vi "Generate3DTest.vi"(8 "error in (no error)":errorcluster, 11 "Local":T6={"Parameter"={"3D Plot"=[], "3D Scatter"=refnum, "Data"={"Split"={"X Train"=[], "X Test"=[], "Y Train"=[], "Y Test"=[]}, "Predict"=[]}, "Display"={"Choice"=enum."All", "Indexe"={"X"=0, "Y"=1, "Z"=2}}, "Point Property"={"Train Style"=enum."Full circle", "Test OK Style"=enum."Full square", "Label Color"=[8978528, 4367871, 1985280], "Test NO OK"={"Style"=enum."Cross", "Color"=16716800}}, "3D Plot Datatype.lvclass"=refnum}, "3DArray"=[], "Rating 3D Array"=[], "GoodPredict"=0, "Point ID"=[]}) -> (0 "error out":errorcluster, 3 "Local Out":T6)   [LabVIEW 2020]
doc: "Generate the 3D graph with preticted data"
uses:
  _Controls/3DParameters.ctl
  <vilib>/Math Plots/3D Math Plots/3D Plot/3D Plot Datatype/3D Plot Datatype.lvclass
  <vilib>/Math Plots/3D Math Plots/3D Scatter/3D Scatter XCtrl/3D Scatter.xctl
  _Controls/Datas.ctl
  _Controls/PointPropertyMultipleLabel.ctl
  _Controls/Style.ctl
  _Controls/3DData.ctl
types:
  T1 = typedef "3DParameters.ctl" = cluster{"3D Plot":refnum<class "3D Plot Datatype.lvclass">[], "3D Scatter":refnum<vi>, "Data":T2, "Display":cluster{"Choice":enum16{"All", "Train", "Test"}, "Indexe":cluster{"X":i32, "Y":i32, "Z":i32}}, "Point Property":T3, "3D Plot Datatype.lvclass":refnum<class "3D Plot Datatype.lvclass">}
  T2 = typedef "Datas.ctl" = cluster{"Split":cluster{"X Train":dbl[][], "X Test":dbl[][], "Y Train":dbl[][], "Y Test":dbl[][]}, "Predict":dbl[][]}
  T3 = typedef "PointPropertyMultipleLabel.ctl" = cluster{"Train Style":T4, "Test OK Style":T4, "Label Color":u32[], "Test NO OK":cluster{"Style":T4, "Color":u32}}
  T4 = typedef "Style.ctl" = enum16{"Empty circle", "Full circle", "Empty square", "Full square", "Cross"}
  T5 = typedef "3DData.ctl" = cluster{"Tag":i32, "X":dbl[], "Y":dbl[], "Z":dbl[]}
  T6 = cluster{"Parameter":T1, "3DArray":cluster{"X":dbl[], "Y":dbl[], "Z":dbl[]}[], "Rating 3D Array":T5[], "GoodPredict":i32, "Point ID":cluster{"DataUse":enum16{"Dataset", "Train", "Test"}, "Color":u32}[]}
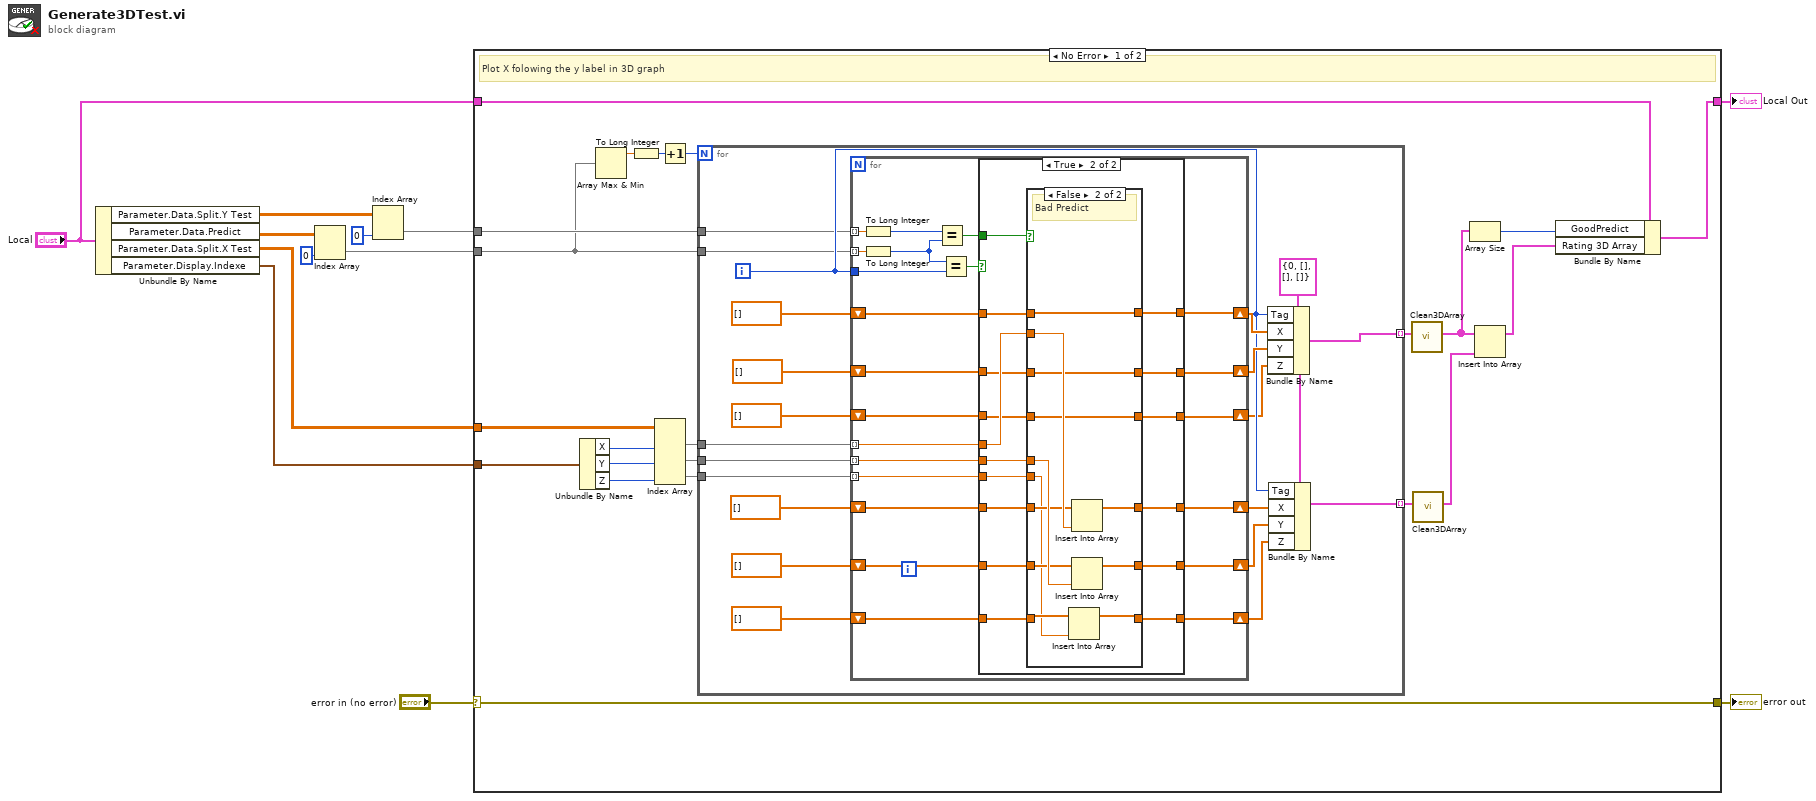
[diagram p0: block diagram]
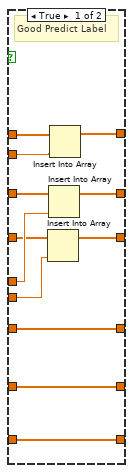
[diagram p3: hidden frame]
diagram:
  n1 = Unbundle By Name("Local") -> ("Parameter.Data.Split.Y Test"=w8:dbl[][], "Parameter.Data.Predict"=w9:dbl[][], "Parameter.Data.Split.X Test"=w5:dbl[][], "Parameter.Display.Indexe"=w3:cluster{"X":i32, "Y":i32, "Z":i32})
  n2 = Index Array(array=w9, index (col)=0 ("disabled index (col)")) -> (element=w6:dbl[])  [unwired: 1 in]
  n3 = Index Array(array=w8, index (col)=0 ("disabled index (col)")) -> (element=w7:dbl[])  [unwired: 1 in]
  n4 = case shown="No Error" "error in (no error)" {
    selector: "error in (no error)" -> [w14 w125]
    tunnel: w5 -> [w32 _]
    tunnel: w6 -> [w24 _]
    tunnel: [w14 w125] -> w12
    tunnel: w7 -> [w25 _]
    tunnel: "Local" -> [w29 w124]
    tunnel: [w28 w124] -> w1
    tunnel: w3 -> [w27 _]
    frame No Error {
      # "Plot X folowing the y label in 3D graph"
      n5 = Unbundle By Name(w27) -> ("X"=w31:i32, "Y"=w30:i32, "Z"=w26:i32)
      n6 = Array Max & Min(array=w24) -> (max value=w34:dbl)  [unwired: 3 out]
      n7 = To Long Integer(number=w34) -> (32bit integer=w33:i32)
      n8 = Index Array(array=w32, index (col) #1=w31, index (col) #2=w30, index (col) #3=w26) -> (element #1=w22:dbl[], element #2=w21:dbl[], element #3=w20:dbl[])  [unwired: 3 in]
      n9 = Increment(x=w33) -> (x+1=w23:i32)
      n10 = for {
        N: w23 -> [_]
        tunnel: w22 -> [w43]
        tunnel: w21 -> [w55]
        tunnel: w24 -> [w41]
        tunnel: [w52] -> w18 mode=indexing
        tunnel: w25 -> [w42]
        tunnel: [w47] -> w16 mode=indexing
        tunnel: w20 -> [w39]
        i -> [w44]
        w35 = T5 {"Tag"=0, "X"=[], "Y"=[], "Z"=[]} ("3D Data")
        n11 = for {
          tunnel: w41 -> [w77] mode=indexing
          tunnel: w43 -> [w76] mode=indexing
          tunnel: w55 -> [w75] mode=indexing
          shift-right: [w73] -> w54
          shift-left: dbl[] [] -> [w72]
          shift-right: [w74] -> w53
          shift-left: dbl[] [] -> [w71]
          tunnel: w44 -> [w70]
          tunnel: w42 -> [w68] mode=indexing
          shift-right: [w61] -> w45
          shift-left: dbl[] [] -> [w63]
          shift-right: [w62] -> w46
          shift-left: dbl[] [] -> [w64]
          shift-right: [w60] -> w36
          shift-left: dbl[] [] -> [w59]
          tunnel: w39 -> [w58] mode=indexing
          shift-right: [w56] -> w37
          shift-left: dbl[] [] -> [w57]
          n12 = To Long Integer(number=w68) -> (32bit integer=w67:i32)
          n13 = To Long Integer(number=w77) -> (32bit integer=w65:i32)
          n14 = Equal?(x=w67, y=w65) -> (x = y?=w66:bool)
          n15 = Equal?(x=w65, y=w70) -> (x = y?=w69:bool)
          n16 = case shown="True" w69 {
            tunnel: w76 -> [_ w98]
            tunnel: w75 -> [_ w94]
            tunnel: [w82 w96] -> w74
            tunnel: [w83 w97] -> w73
            tunnel: w72 -> [w83 w99]
            tunnel: w71 -> [w82 w95]
            tunnel: w66 -> [_ w93]
            tunnel: w63 -> [w80 w90]
            tunnel: w64 -> [w81 w92]
            tunnel: [w81 w91] -> w62
            tunnel: [w80 w89] -> w61
            tunnel: w59 -> [w78 w87]
            tunnel: [w78 w88] -> w60
            tunnel: w58 -> [_ w86]
            tunnel: [w79 w84] -> w56
            tunnel: w57 -> [w79 w85]
            frame False {
            }
            frame True {
              n17 = case shown="False" w93 {
                tunnel: w99 -> [w111 w117]
                tunnel: w98 -> [w110 w123]
                tunnel: [w109 w117] -> w97
                tunnel: [w108 w118] -> w96
                tunnel: w95 -> [w107 w118]
                tunnel: w94 -> [w106 w122]
                tunnel: w92 -> [w104 w121]
                tunnel: [w104 w116] -> w91
                tunnel: w90 -> [w105 w120]
                tunnel: [w105 w119] -> w89
                tunnel: w87 -> [w103 w115]
                tunnel: [w103 w114] -> w88
                tunnel: w86 -> [w100 w113]
                tunnel: [w101 w112] -> w84
                tunnel: w85 -> [w102 w112]
                frame True {
                  # "Good Predict Label"
                  n18 = Insert Into Array(array=w102, new element=w100) -> (w101:dbl[])  [unwired: 1 in]
                  n19 = Insert Into Array(array=w107, new element=w106) -> (w108:dbl[])  [unwired: 1 in]
                  n20 = Insert Into Array(array=w111, new element=w110) -> (w109:dbl[])  [unwired: 1 in]
                }
                frame False {
                  # "Bad Predict"
                  n21 = Insert Into Array(array=w115, new element=w113) -> (w114:dbl[])  [unwired: 1 in]
                  n22 = Insert Into Array(array=w120, new element=w123) -> (w119:dbl[])  [unwired: 1 in]
                  n23 = Insert Into Array(array=w121, new element=w122) -> (w116:dbl[])  [unwired: 1 in]
                }
              }
            }
          }
        }
        n24 = Bundle By Name(cluster=w35, "Tag"=w44, "X"=w54, "Y"=w53, "Z"=w37) -> (w52:T5)
        n25 = Bundle By Name(cluster=w35, "Tag"=w44, "X"=w45, "Y"=w46, "Z"=w36) -> (w47:T5)
      }
      n26 = call "Clean3DArray.vi"("3D Array"=w18) -> ("Array3DClean"=w17:T5[])  [unwired: 10 in]
      n27 = call "Clean3DArray.vi"("3D Array"=w16) -> ("Array3DClean"=w15:T5[])  [unwired: 10 in]
      n28 = Array Size(array=w17) -> (size(s)=w13:i32)
      n29 = Insert Into Array(array=w17, new element=w15) -> (w19:T5[])  [unwired: 1 in]
      n30 = Bundle By Name(cluster=w29, "GoodPredict"=w13, "Rating 3D Array"=w19) -> (w28:T6)
    }
    frame Error {
    }
  }
  "error out" <- w12
  "Local Out" <- w1
